vi "FipsAdjacent.vi"() -> (11 "Fips":i32[](array[numeric]))   [LabVIEW 2017] (continued)
KS\"\t20097\t\"Ford County, KS\"\t20057\n\"Kiowa County, KS\"\t20097\t\"Kiowa County, KS\"\t20097\n\"Kiowa County, KS\"\t20097\t\"Pratt County, KS\"\t20151\n\"Labette County, KS\"\t20099\t\"Cherokee County, KS\"\t20021\n\"Labette County, KS\"\t20099\t\"Crawford County, KS\"\t20037\n\"Labette County, KS\"\t20099\t\"Labette County, KS\"\t20099\n\"Labette County, KS\"\t20099\t\"Montgomery County, KS\"\t20125\n\"Labette County, KS\"\t20099\t\"Neosho County, KS\"\t20133\n\"Labette County, KS\"\t20099\t\"Craig County, OK\"\t40035\n\"Labette County, KS\"\t20099\t\"Nowata County, OK\"\t40105\n\"Lane County, KS\"\t20101\t\"Finney County, KS\"\t20055\n\"Lane County, KS\"\t20101\t\"Gove County, KS\"\t20063\n\"Lane County, KS\"\t20101\t\"Lane County, KS\"\t20101\n\"Lane County, KS\"\t20101\t\"Ness County, KS\"\t20135\n\"Lane County, KS\"\t20101\t\"Scott County, KS\"\t20171\n\"Leavenworth County, KS\"\t20103\t\"Atchison County, KS\"\t20005\n\"Leavenworth County, KS\"\t20103\t\"Douglas County, KS\"\t20045\n\"Leavenworth County, KS\"\t20103\t\"Jefferson County, KS\"\t20087\n\"Leavenworth County, KS\"\t20103\t\"Johnson County, KS\"\t20091\n\"Leavenworth County, KS\"\t20103\t\"Leavenworth County, KS\"\t20103\n\"Leavenworth County, KS\"\t20103\t\"Wyandotte County, KS\"\t20209\n\"Leavenworth County, KS\"\t20103\t\"Platte County, MO\"\t29165\n\"Lincoln County, KS\"\t20105\t\"Ellsworth County, KS\"\t20053\n\"Lincoln County, KS\"\t20105\t\"Lincoln County, KS\"\t20105\n\"Lincoln County, KS\"\t20105\t\"Mitchell County, KS\"\t20123\n\"Lincoln County, KS\"\t20105\t\"Osborne County, KS\"\t20141\n\"Lincoln County, KS\"\t20105\t\"Ottawa County, KS\"\t20143\n\"Lincoln County, KS\"\t20105\t\"Russell County, KS\"\t20167\n\"Lincoln County, KS\"\t20105\t\"Saline County, KS\"\t20169\n\"Linn County, KS\"\t20107\t\"Allen County, KS\"\t20001\n\"Linn County, KS\"\t20107\t\"Anderson County, KS\"\t20003\n\"Linn County, KS\"\t20107\t\"Bourbon County, KS\"\t20011\n\"Linn County, KS\"\t20107\t\"Franklin County, KS\"\t20059\n\"Linn County, KS\"\t20107\t\"Linn County, KS\"\t20107\n\"Linn County, KS\"\t20107\t\"Miami County, KS\"\t20121\n\"Linn County, KS\"\t20107\t\"Bates County, MO\"\t29013\n\"Linn County, KS\"\t20107\t\"Vernon County, MO\"\t29217\n\"Logan County, KS\"\t20109\t\"Gove County, KS\"\t20063\n\"Logan County, KS\"\t20109\t\"Logan County, KS\"\t20109\n\"Logan County, KS\"\t20109\t\"Scott County, KS\"\t20171\n\"Logan County, KS\"\t20109\t\"Sherman County, KS\"\t20181\n\"Logan County, KS\"\t20109\t\"Thomas County, KS\"\t20193\n\"Logan County, KS\"\t20109\t\"Wallace County, KS\"\t20199\n\"Logan County, KS\"\t20109\t\"Wichita County, KS\"\t20203\n\"Lyon County, KS\"\t20111\t\"Chase County, KS\"\t20017\n\"Lyon County, KS\"\t20111\t\"Coffey County, KS\"\t20031\n\"Lyon County, KS\"\t20111\t\"Greenwood County, KS\"\t20073\n\"Lyon County, KS\"\t20111\t\"Lyon County, KS\"\t20111\n\"Lyon County, KS\"\t20111\t\"Morris County, KS\"\t20127\n\"Lyon County, KS\"\t20111\t\"Osage County, KS\"\t20139\n\"Lyon County, KS\"\t20111\t\"Wabaunsee County, KS\"\t20197\n\"McPherson County, KS\"\t20113\t\"Dickinson County, KS\"\t20041\n\"McPherson County, KS\"\t20113\t\"Ellsworth County, KS\"\t20053\n\"McPherson County, KS\"\t20113\t\"Harvey County, KS\"\t20079\n\"McPherson County, KS\"\t20113\t\"McPherson County, KS\"\t20113\n\"McPherson County, KS\"\t20113\t\"Marion County, KS\"\t20115\n\"McPherson County, KS\"\t20113\t\"Reno County, KS\"\t20155\n\"McPherson County, KS\"\t20113\t\"Rice County, KS\"\t20159\n\"McPherson County, KS\"\t20113\t\"Saline County, KS\"\t20169\n\"Marion County, KS\"\t20115\t\"Butler County, KS\"\t20015\n\"Marion County, KS\"\t20115\t\"Chase County, KS\"\t20017\n\"Marion County, KS\"\t20115\t\"Dickinson County, KS\"\t20041\n\"Marion County, KS\"\t20115\t\"Harvey County, KS\"\t20079\n\"Marion County, KS\"\t20115\t\"McPherson County, KS\"\t20113\n\"Marion County, KS\"\t20115\t\"Marion County, KS\"\t20115\n\"Marion County, KS\"\t20115\t\"Morris County, KS\"\t20127\n\"Marion County, KS\"\t20115\t\"Saline County, KS\"\t20169\n\"Marshall County, KS\"\t20117\t\"Marshall County, KS\"\t20117\n\"Marshall County, KS\"\t20117\t\"Nemaha County, KS\"\t20131\n\"Marshall County, KS\"\t20117\t\"Pottawatomie County, KS\"\t20149\n\"Marshall County, KS\"\t20117\t\"Riley County, KS\"\t20161\n\"Marshall County, KS\"\t20117\t\"Washington County, KS\"\t20201\n\"Marshall County, KS\"\t20117\t\"Gage County, NE\"\t31067\n\"Marshall County, KS\"\t20117\t\"Pawnee County, NE\"\t31133\n\"Meade County, KS\"\t20119\t\"Clark County, KS\"\t20025\n\"Meade County, KS\"\t20119\t\"Ford County, KS\"\t20057\n\"Meade County, KS\"\t20119\t\"Gray County, KS\"\t20069\n\"Meade County, KS\"\t20119\t\"Haskell County, KS\"\t20081\n\"Meade County, KS\"\t20119\t\"Meade County, KS\"\t20119\n\"Meade County, KS\"\t20119\t\"Seward County, KS\"\t20175\n\"Meade County, KS\"\t20119\t\"Beaver County, OK\"\t40007\n\"Miami County, KS\"\t20121\t\"Anderson County, KS\"\t20003\n\"Miami County, KS\"\t20121\t\"Douglas County, KS\"\t20045\n\"Miami County, KS\"\t20121\t\"Franklin County, KS\"\t20059\n\"Miami County, KS\"\t20121\t\"Johnson County, KS\"\t20091\n\"Miami County, KS\"\t20121\t\"Linn County, KS\"\t20107\n\"Miami County, KS\"\t20121\t\"Miami County, KS\"\t20121\n\"Miami County, KS\"\t20121\t\"Bates County, MO\"\t29013\n\"Miami County, KS\"\t20121\t\"Cass County, MO\"\t29037\n\"Mitchell County, KS\"\t20123\t\"Cloud County, KS\"\t20029\n\"Mitchell County, KS\"\t20123\t\"Jewell County, KS\"\t20089\n\"Mitchell County, KS\"\t20123\t\"Lincoln County, KS\"\t20105\n\"Mitchell County, KS\"\t20123\t\"Mitchell County, KS\"\t20123\n\"Mitchell County, KS\"\t20123\t\"Osborne County, KS\"\t20141\n\"Mitchell County, KS\"\t20123\t\"Ottawa County, KS\"\t20143\n\"Montgomery County, KS\"\t20125\t\"Chautauqua County, KS\"\t20019\n\"Montgomery County, KS\"\t20125\t\"Elk County, KS\"\t20049\n\"Montgomery County, KS\"\t20125\t\"Labette County, KS\"\t20099\n\"Montgomery County, KS\"\t20125\t\"Montgomery County, KS\"\t20125\n\"Montgomery County, KS\"\t20125\t\"Neosho County, KS\"\t20133\n\"Montgomery County, KS\"\t20125\t\"Wilson County, KS\"\t20205\n\"Montgomery County, KS\"\t20125\t\"Nowata County, OK\"\t40105\n\"Montgomery County, KS\"\t20125\t\"Washington County, OK\"\t40147\n\"Morris County, KS\"\t20127\t\"Chase County, KS\"\t20017\n\"Morris County, KS\"\t20127\t\"Dickinson County, KS\"\t20041\n\"Morris County, KS\"\t20127\t\"Geary County, KS\"\t20061\n\"Morris County, KS\"\t20127\t\"Lyon County, KS\"\t20111\n\"Morris County, KS\"\t20127\t\"Marion County, KS\"\t20115\n\"Morris County, KS\"\t20127\t\"Morris County, KS\"\t20127\n\"Morris County, KS\"\t20127\t\"Wabaunsee County, KS\"\t20197\n\"Morton County, KS\"\t20129\t\"Baca County, CO\"\t08009\n\"Morton County, KS\"\t20129\t\"Morton County, KS\"\t20129\n\"Morton County, KS\"\t20129\t\"Stanton County, KS\"\t20187\n\"Morton County, KS\"\t20129\t\"Stevens County, KS\"\t20189\n\"Morton County, KS\"\t20129\t\"Cimarron County, OK\"\t40025\n\"Morton County, KS\"\t20129\t\"Texas County, OK\"\t40139\n\"Nemaha County, KS\"\t20131\t\"Brown County, KS\"\t20013\n\"Nemaha County, KS\"\t20131\t\"Jackson County, KS\"\t20085\n\"Nemaha County, KS\"\t20131\t\"Marshall County, KS\"\t20117\n\"Nemaha County, KS\"\t20131\t\"Nemaha County, KS\"\t20131\n\"Nemaha County, KS\"\t20131\t\"Pottawatomie County, KS\"\t20149\n\"Nemaha County, KS\"\t20131\t\"Pawnee County, NE\"\t31133\n\"Nemaha County, KS\"\t20131\t\"Richardson County, NE\"\t31147\n\"Neosho County, KS\"\t20133\t\"Allen County, KS\"\t20001\n\"Neosho County, KS\"\t20133\t\"Bourbon County, KS\"\t20011\n\"Neosho County, KS\"\t20133\t\"Crawford County, KS\"\t20037\n\"Neosho County, KS\"\t20133\t\"Labette County, KS\"\t20099\n\"Neosho County, KS\"\t20133\t\"Montgomery County, KS\"\t20125\n\"Neosho County, KS\"\t20133\t\"Neosho County, KS\"\t20133\n\"Neosho County, KS\"\t20133\t\"Wilson County, KS\"\t20205\n\"Neosho County, KS\"\t20133\t\"Woodson County, KS\"\t20207\n\"Ness County, KS\"\t20135\t\"Ellis County, KS\"\t20051\n\"Ness County, KS\"\t20135\t\"Finney County, KS\"\t20055\n\"Ness County, KS\"\t20135\t\"Gove County, KS\"\t20063\n\"Ness County, KS\"\t20135\t\"Hodgeman County, KS\"\t20083\n\"Ness County, KS\"\t20135\t\"Lane County, KS\"\t20101\n\"Ness County, KS\"\t20135\t\"Ness County, KS\"\t20135\n\"Ness County, KS\"\t20135\t\"Pawnee County, KS\"\t20145\n\"Ness County, KS\"\t20135\t\"Rush County, KS\"\t20165\n\"Ness County, KS\"\t20135\t\"Trego County, KS\"\t20195\n\"Norton County, KS\"\t20137\t\"Decatur County, KS\"\t20039\n\"Norton County, KS\"\t20137\t\"Graham County, KS\"\t20065\n\"Norton County, KS\"\t20137\t\"Norton County, KS\"\t20137\n\"Norton County, KS\"\t20137\t\"Phillips County, KS\"\t20147\n\"Norton County, KS\"\t20137\t\"Sheridan County, KS\"\t20179\n\"Norton County, KS\"\t20137\t\"Furnas County, NE\"\t31065\n\"Norton County, KS\"\t20137\t\"Harlan County, NE\"\t31083\n\"Osage County, KS\"\t20139\t\"Coffey County, KS\"\t20031\n\"Osage County, KS\"\t20139\t\"Douglas County, KS\"\t20045\n\"Osage County, KS\"\t20139\t\"Franklin County, KS\"\t20059\n\"Osage County, KS\"\t20139\t\"Lyon County, KS\"\t20111\n\"Osage County, KS\"\t20139\t\"Osage County, KS\"\t20139\n\"Osage County, KS\"\t20139\t\"Shawnee County, KS\"\t20177\n\"Osage County, KS\"\t20139\t\"Wabaunsee County, KS\"\t20197\n\"Osborne County, KS\"\t20141\t\"Ellis County, KS\"\t20051\n\"Osborne County, KS\"\t20141\t\"Jewell County, KS\"\t20089\n\"Osborne County, KS\"\t20141\t\"Lincoln County, KS\"\t20105\n\"Osborne County, KS\"\t20141\t\"Mitchell County, KS\"\t20123\n\"Osborne County, KS\"\t20141\t\"Osborne County, KS\"\t20141\n\"Osborne County, KS\"\t20141\t\"Rooks County, KS\"\t20163\n\"Osborne County, KS\"\t20141\t\"Russell County, KS\"\t20167\n\"Osborne County, KS\"\t20141\t\"Smith County, KS\"\t20183\n\"Ottawa County, KS\"\t20143\t\"Clay County, KS\"\t20027\n\"Ottawa County, KS\"\t20143\t\"Cloud County, KS\"\t20029\n\"Ottawa County, KS\"\t20143\t\"Dickinson County, KS\"\t20041\n\"Ottawa County, KS\"\t20143\t\"Lincoln County, KS\"\t20105\n\"Ottawa County, KS\"\t20143\t\"Mitchell County, KS\"\t20123\n\"Ottawa County, KS\"\t20143\t\"Ottawa County, KS\"\t20143\n\"Ottawa County, KS\"\t20143\t\"Saline County, KS\"\t20169\n\"Pawnee County, KS\"\t20145\t\"Barton County, KS\"\t20009\n\"Pawnee County, KS\"\t20145\t\"Edwards County, KS\"\t20047\n\"Pawnee County, KS\"\t20145\t\"Hodgeman County, KS\"\t20083\n\"Pawnee County, KS\"\t20145\t\"Ness County, KS\"\t20135\n\"Pawnee County, KS\"\t20145\t\"Pawnee County, KS\"\t20145\n\"Pawnee County, KS\"\t20145\t\"Rush County, KS\"\t20165\n\"Pawnee County, KS\"\t20145\t\"Stafford County, KS\"\t20185\n\"Phillips County, KS\"\t20147\t\"Graham County, KS\"\t20065\n\"Phillips County, KS\"\t20147\t\"Norton County, KS\"\t20137\n\"Phillips County, KS\"\t20147\t\"Phillips County, KS\"\t20147\n\"Phillips County, KS\"\t20147\t\"Rooks County, KS\"\t20163\n\"Phillips County, KS\"\t20147\t\"Smith County, KS\"\t20183\n\"Phillips County, KS\"\t20147\t\"Franklin County, NE\"\t31061\n\"Phillips County, KS\"\t20147\t\"Harlan County, NE\"\t31083\n\"Pottawatomie County, KS\"\t20149\t\"Jackson County, KS\"\t20085\n\"Pottawatomie County, KS\"\t20149\t\"Marshall County, KS\"\t20117\n\"Pottawatomie County, KS\"\t20149\t\"Nemaha County, KS\"\t20131\n\"Pottawatomie County, KS\"\t20149\t\"Pottawatomie County, KS\"\t20149\n\"Pottawatomie County, KS\"\t20149\t\"Riley County, KS\"\t20161\n\"Pottawatomie County, KS\"\t20149\t\"Shawnee County, KS\"\t20177\n\"Pottawatomie County, KS\"\t20149\t\"Wabaunsee County, KS\"\t20197\n\"Pratt County, KS\"\t20151\t\"Barber County, KS\"\t20007\n\"Pratt County, KS\"\t20151\t\"Edwards County, KS\"\t20047\n\"Pratt County, KS\"\t20151\t\"Kingman County, KS\"\t20095\n\"Pratt County, KS\"\t20151\t\"Kiowa County, KS\"\t20097\n\"Pratt County, KS\"\t20151\t\"Pratt County, KS\"\t20151\n\"Pratt County, KS\"\t20151\t\"Reno County, KS\"\t20155\n\"Pratt County, KS\"\t20151\t\"Stafford County, KS\"\t20185\n\"Rawlins County, KS\"\t20153\t\"Cheyenne County, KS\"\t20023\n\"Rawlins County, KS\"\t20153\t\"Decatur County, KS\"\t20039\n\"Rawlins County, KS\"\t20153\t\"Rawlins County, KS\"\t20153\n\"Rawlins County, KS\"\t20153\t\"Sherman County, KS\"\t20181\n\"Rawlins County, KS\"\t20153\t\"Thomas County, KS\"\t20193\n\"Rawlins County, KS\"\t20153\t\"Dundy County, NE\"\t31057\n\"Rawlins County, KS\"\t20153\t\"Hitchcock County, NE\"\t31087\n\"Rawlins County, KS\"\t20153\t\"Red Willow County, NE\"\t31145\n\"Reno County, KS\"\t20155\t\"Harvey County, KS\"\t20079\n\"Reno County, KS\"\t20155\t\"Kingman County, KS\"\t20095\n\"Reno County, KS\"\t20155\t\"McPherson County, KS\"\t20113\n\"Reno County, KS\"\t20155\t\"Pratt County, KS\"\t20151\n\"Reno County, KS\"\t20155\t\"Reno County, KS\"\t20155\n\"Reno County, KS\"\t20155\t\"Rice County, KS\"\t20159\n\"Reno County, KS\"\t20155\t\"Sedgwick County, KS\"\t20173\n\"Reno County, KS\"\t20155\t\"Stafford County, KS\"\t20185\n\"Republic County, KS\"\t20157\t\"Cloud County, KS\"\t20029\n\"Republic County, KS\"\t20157\t\"Jewell County, KS\"\t20089\n\"Republic County, KS\"\t20157\t\"Republic County, KS\"\t20157\n\"Republic County, KS\"\t20157\t\"Washington County, KS\"\t20201\n\"Republic County, KS\"\t20157\t\"Jefferson County, NE\"\t31095\n\"Republic County, KS\"\t20157\t\"Nuckolls County, NE\"\t31129\n\"Republic County, KS\"\t20157\t\"Thayer County, NE\"\t31169\n\"Rice County, KS\"\t20159\t\"Barton County, KS\"\t20009\n\"Rice County, KS\"\t20159\t\"Ellsworth County, KS\"\t20053\n\"Rice County, KS\"\t20159\t\"McPherson County, KS\"\t20113\n\"Rice County, KS\"\t20159\t\"Reno County, KS\"\t20155\n\"Rice County, KS\"\t20159\t\"Rice County, KS\"\t20159\n\"Rice County, KS\"\t20159\t\"Stafford County, KS\"\t20185\n\"Riley County, KS\"\t20161\t\"Clay County, KS\"\t20027\n\"Riley County, KS\"\t20161\t\"Geary County, KS\"\t20061\n\"Riley County, KS\"\t20161\t\"Marshall County, KS\"\t20117\n\"Riley County, KS\"\t20161\t\"Pottawatomie County, KS\"\t20149\n\"Riley County, KS\"\t20161\t\"Riley County, KS\"\t20161\n\"Riley County, KS\"\t20161\t\"Wabaunsee County, KS\"\t20197\n\"Riley County, KS\"\t20161\t\"Washington County, KS\"\t20201\n\"Rooks County, KS\"\t20163\t\"Ellis County, KS\"\t20051\n\"Rooks County, KS\"\t20163\t\"Graham County, KS\"\t20065\n\"Rooks County, KS\"\t20163\t\"Osborne County, KS\"\t20141\n\"Rooks County, KS\"\t20163\t\"Phillips County, KS\"\t20147\n\"Rooks County, KS\"\t20163\t\"Rooks County, KS\"\t20163\n\"Rooks County, KS\"\t20163\t\"Smith County, KS\"\t20183\n\"Rooks County, KS\"\t20163\t\"Trego County, KS\"\t20195\n\"Rush County, KS\"\t20165\t\"Barton County, KS\"\t20009\n\"Rush County, KS\"\t20165\t\"Ellis County, KS\"\t20051\n\"Rush County, KS\"\t20165\t\"Ness County, KS\"\t20135\n\"Rush County, KS\"\t20165\t\"Pawnee County, KS\"\t20145\n\"Rush County, KS\"\t20165\t\"Rush County, KS\"\t20165\n\"Rush County, KS\"\t20165\t\"Russell County, KS\"\t20167\n\"Russell County, KS\"\t20167\t\"Barton County, KS\"\t20009\n\"Russell County, KS\"\t20167\t\"Ellis County, KS\"\t20051\n\"Russell County, KS\"\t20167\t\"Ellsworth County, KS\"\t20053\n\"Russell County, KS\"\t20167\t\"Lincoln County, KS\"\t20105\n\"Russell County, KS\"\t20167\t\"Osborne County, KS\"\t20141\n\"Russell County, KS\"\t20167\t\"Rush County, KS\"\t20165\n\"Russell County, KS\"\t20167\t\"Russell County, KS\"\t20167\n\"Saline County, KS\"\t20169\t\"Dickinson County, KS\"\t20041\n\"Saline County, KS\"\t20169\t\"Ellsworth County, KS\"\t20053\n\"Saline County, KS\"\t20169\t\"Lincoln County, KS\"\t20105\n\"Saline County, KS\"\t20169\t\"McPherson County, KS\"\t20113\n\"Saline County, KS\"\t20169\t\"Marion County, KS\"\t20115\n\"Saline County, KS\"\t20169\t\"Ottawa County, KS\"\t20143\n\"Saline County, KS\"\t20169\t\"Saline County, KS\"\t20169\n\"Scott County, KS\"\t20171\t\"Finney County, KS\"\t20055\n\"Scott County, KS\"\t20171\t\"Gove County, KS\"\t20063\n\"Scott County, KS\"\t20171\t\"Kearny County, KS\"\t20093\n\"Scott County, KS\"\t20171\t\"Lane County, KS\"\t20101\n\"Scott County, KS\"\t20171\t\"Logan County, KS\"\t20109\n\"Scott County, KS\"\t20171\t\"Scott County, KS\"\t20171\n\"Scott County, KS\"\t20171\t\"Wichita County, KS\"\t20203\n\"Sedgwick County, KS\"\t20173\t\"Butler County, KS\"\t20015\n\"Sedgwick County, KS\"\t20173\t\"Cowley County, KS\"\t20035\n\"Sedgwick County, KS\"\t20173\t\"Harvey County, KS\"\t20079\n\"Sedgwick County, KS\"\t20173\t\"Kingman County, KS\"\t20095\n\"Sedgwick County, KS\"\t20173\t\"Reno County, KS\"\t20155\n\"Sedgwick County, KS\"\t20173\t\"Sedgwick County, KS\"\t20173\n\"Sedgwick County, KS\"\t20173\t\"Sumner County, KS\"\t20191\n\"Seward County, KS\"\t20175\t\"Haskell County, KS\"\t20081\n\"Seward County, KS\"\t20175\t\"Meade County, KS\"\t20119\n\"Seward County, KS\"\t20175\t\"Seward County, KS\"\t20175\n\"Seward County, KS\"\t20175\t\"Stevens County, KS\"\t20189\n\"Seward County, KS\"\t20175\t\"Beaver County, OK\"\t40007\n\"Seward County, KS\"\t20175\t\"Texas County, OK\"\t40139\n\"Shawnee County, KS\"\t20177\t\"Douglas County, KS\"\t20045\n\"Shawnee County, KS\"\t20177\t\"Jackson County, KS\"\t20085\n\"Shawnee County, KS\"\t20177\t\"Jefferson County, KS\"\t20087\n\"Shawnee County, KS\"\t20177\t\"Osage County, KS\"\t20139\n\"Shawnee County, KS\"\t20177\t\"Pottawatomie County, KS\"\t20149\n\"Shawnee County, KS\"\t20177\t\"Shawnee County, KS\"\t20177\n\"Shawnee County, KS\"\t20177\t\"Wabaunsee County, KS\"\t20197\n\"Sheridan County, KS\"\t20179\t\"Decatur County, KS\"\t20039\n\"Sheridan County, KS\"\t20179\t\"Gove County, KS\"\t20063\n\"Sheridan County, KS\"\t20179\t\"Graham County, KS\"\t20065\n\"Sheridan County, KS\"\t20179\t\"Norton County, KS\"\t20137\n\"Sheridan County, KS\"\t20179\t\"Sheridan County, KS\"\t20179\n\"Sheridan County, KS\"\t20179\t\"Thomas County, KS\"\t20193\n\"Sherman County, KS\"\t20181\t\"Kit Carson County, CO\"\t08063\n\"Sherman County, KS\"\t20181\t\"Cheyenne County, KS\"\t20023\n\"Sherman County, KS\"\t20181\t\"Logan County, KS\"\t20109\n\"Sherman County, KS\"\t20181\t\"Rawlins County, KS\"\t20153\n\"Sherman County, KS\"\t20181\t\"Sherman County, KS\"\t20181\n\"Sherman County, KS\"\t20181\t\"Thomas County, KS\"\t20193\n\"Sherman County, KS\"\t20181\t\"Wallace County, KS\"\t20199\n\"Smith County, KS\"\t20183\t\"Jewell County, KS\"\t20089\n\"Smith County, KS\"\t20183\t\"Osborne County, KS\"\t20141\n\"Smith County, KS\"\t20183\t\"Phillips County, KS\"\t20147\n\"Smith County, KS\"\t20183\t\"Rooks County, KS\"\t20163\n\"Smith County, KS\"\t20183\t\"Smith County, KS\"\t20183\n\"Smith County, KS\"\t20183\t\"Franklin County, NE\"\t31061\n\"Smith County, KS\"\t20183\t\"Webster County, NE\"\t31181\n\"Stafford County, KS\"\t20185\t\"Barton County, KS\"\t20009\n\"Stafford County, KS\"\t20185\t\"Edwards County, KS\"\t20047\n\"Stafford County, KS\"\t20185\t\"Pawnee County, KS\"\t20145\n\"Stafford County, KS\"\t20185\t\"Pratt County, KS\"\t20151\n\"Stafford County, KS\"\t20185\t\"Reno County, KS\"\t20155\n\"Stafford County, KS\"\t20185\t\"Rice County, KS\"\t20159\n\"Stafford County, KS\"\t20185\t\"Stafford County, KS\"\t20185\n\"Stanton County, KS\"\t20187\t\"Baca County, CO\"\t08009\n\"Stanton County, KS\"\t20187\t\"Prowers County, CO\"\t08099\n\"Stanton County, KS\"\t20187\t\"Grant County, KS\"\t20067\n\"Stanton County, KS\"\t20187\t\"Hamilton County, KS\"\t20075\n\"Stanton County, KS\"\t20187\t\"Kearny County, KS\"\t20093\n\"Stanton County, KS\"\t20187\t\"Morton County, KS\"\t20129\n\"Stanton County, KS\"\t20187\t\"Stanton County, KS\"\t20187\n\"Stanton County, KS\"\t20187\t\"Stevens County, KS\"\t20189\n\"Stevens County, KS\"\t20189\t\"Grant County, KS\"\t20067\n\"Stevens County, KS\"\t20189\t\"Haskell County, KS\"\t20081\n\"Stevens County, KS\"\t20189\t\"Morton County, KS\"\t20129\n\"Stevens County, KS\"\t20189\t\"Seward County, KS\"\t20175\n\"Stevens County, KS\"\t20189\t\"Stanton County, KS\"\t20187\n\"Stevens County, KS\"\t20189\t\"Stevens County, KS\"\t20189\n\"Stevens County, KS\"\t20189\t\"Texas County, OK\"\t40139\n\"Sumner County, KS\"\t20191\t\"Butler County, KS\"\t20015\n\"Sumner County, KS\"\t20191\t\"Cowley County, KS\"\t20035\n\"Sumner County, KS\"\t20191\t\"Harper County, KS\"\t20077\n\"Sumner County, KS\"\t20191\t\"Kingman County, KS\"\t20095\n\"Sumner County, KS\"\t20191\t\"Sedgwick County, KS\"\t20173\n\"Sumner County, KS\"\t20191\t\"Sumner County, KS\"\t20191\n\"Sumner County, KS\"\t20191\t\"Grant County, OK\"\t40053\n\"Sumner County, KS\"\t20191\t\"Kay County, OK\"\t40071\n\"Thomas County, KS\"\t20193\t\"Decatur County, KS\"\t20039\n\"Thomas County, KS\"\t20193\t\"Gove County, KS\"\t20063\n\"Thomas County, KS\"\t20193\t\"Logan County, KS\"\t20109\n\"Thomas County, KS\"\t20193\t\"Rawlins County, KS\"\t20153\n\"Thomas County, KS\"\t20193\t\"Sheridan County, KS\"\t20179\n\"Thomas County, KS\"\t20193\t\"Sherman County, KS\"\t20181\n\"Thomas County, KS\"\t20193\t\"Thomas County, KS\"\t20193\n\"Trego County, KS\"\t20195\t\"Ellis County, KS\"\t20051\n\"Trego County, KS\"\t20195\t\"Gove County, KS\"\t20063\n\"Trego County, KS\"\t20195\t\"Graham County, KS\"\t20065\n\"Trego County, KS\"\t20195\t\"Ness County, KS\"\t20135\n\"Trego County, KS\"\t20195\t\"Rooks County, KS\"\t20163\n\"Trego County, KS\"\t20195\t\"Trego County, KS\"\t20195\n\"Wabaunsee County, KS\"\t20197\t\"Geary County, KS\"\t20061\n\"Wabaunsee County, KS\"\t20197\t\"Lyon County, KS\"\t20111\n\"Wabaunsee County, KS\"\t20197\t\"Morris County, KS\"\t20127\n\"Wabaunsee County, KS\"\t20197\t\"Osage County, KS\"\t20139\n\"Wabaunsee County, KS\"\t20197\t\"Pottawatomie County, KS\"\t20149\n\"Wabaunsee County, KS\"\t20197\t\"Riley County, KS\"\t20161\n\"Wabaunsee County, KS\"\t20197\t\"Shawnee County, KS\"\t20177\n\"Wabaunsee County, KS\"\t20197\t\"Wabaunsee County, KS\"\t20197\n\"Wallace County, KS\"\t20199\t\"Cheyenne County, CO\"\t08017\n\"Wallace County, KS\"\t20199\t\"Kit Carson County, CO\"\t08063\n\"Wallace County, KS\"\t20199\t\"Greeley County, KS\"\t20071\n\"Wallace County, KS\"\t20199\t\"Logan County, KS\"\t20109\n\"Wallace County, KS\"\t20199\t\"Sherman County, KS\"\t20181\n\"Wallace County, KS\"\t20199\t\"Wallace County, KS\"\t20199\n\"Wallace County, KS\"\t20199\t\"Wichita County, KS\"\t20203\n\"Washington County, KS\"\t20201\t\"Clay County, KS\"\t20027\n\"Washington County, KS\"\t20201\t\"Cloud County, KS\"\t20029\n\"Washington County, KS\"\t20201\t\"Marshall County, KS\"\t20117\n\"Washington County, KS\"\t20201\t\"Republic County, KS\"\t20157\n\"Washington County, KS\"\t20201\t\"Riley County, KS\"\t20161\n\"Washington County, KS\"\t20201\t\"Washington County, KS\"\t20201\n\"Washington County, KS\"\t20201\t\"Gage County, NE\"\t31067\n\"Washington County, KS\"\t20201\t\"Jefferson County, NE\"\t31095\n\"Washington County, KS\"\t20201\t\"Thayer County, NE\"\t31169\n\"Wichita County, KS\"\t20203\t\"Greeley County, KS\"\t20071\n\"Wichita County, KS\"\t20203\t\"Hamilton County, KS\"\t20075\n\"Wichita County, KS\"\t20203\t\"Kearny County, KS\"\t20093\n\"Wichita County, KS\"\t20203\t\"Logan County, KS\"\t20109\n\"Wichita County, KS\"\t20203\t\"Scott County, KS\"\t20171\n\"Wichita County, KS\"\t20203\t\"Wallace County, KS\"\t20199\n\"Wichita County, KS\"\t20203\t\"Wichita County, KS\"\t20203\n\"Wilson County, KS\"\t20205\t\"Allen County, KS\"\t20001\n\"Wilson County, KS\"\t20205\t\"Elk County, KS\"\t20049\n\"Wilson County, KS\"\t20205\t\"Greenwood County, KS\"\t20073\n\"Wilson County, KS\"\t20205\t\"Montgomery County, KS\"\t20125\n\"Wilson County, KS\"\t20205\t\"Neosho County, KS\"\t20133\n\"Wilson County, KS\"\t20205\t\"Wilson County, KS\"\t20205\n\"Wilson County, KS\"\t20205\t\"Woodson County, KS\"\t20207\n\"Woodson County, KS\"\t20207\t\"Allen County, KS\"\t20001\n\"Woodson County, KS\"\t20207\t\"Anderson County, KS\"\t20003\n\"Woodson County, KS\"\t20207\t\"Coffey County, KS\"\t20031\n\"Woodson County, KS\"\t20207\t\"Greenwood County, KS\"\t20073\n\"Woodson County, KS\"\t20207\t\"Neosho County, KS\"\t20133\n\"Woodson County, KS\"\t20207\t\"Wilson County, KS\"\t20205\n\"Woodson County, KS\"\t20207\t\"Woodson County, KS\"\t20207\n\"Wyandotte County, KS\"\t20209\t\"Johnson County, KS\"\t20091\n\"Wyandotte County, KS\"\t20209\t\"Leavenworth County, KS\"\t20103\n\"Wyandotte County, KS\"\t20209\t\"Wyandotte County, KS\"\t20209\n\"Wyandotte County, KS\"\t20209\t\"Clay County, MO\"\t29047\n\"Wyandotte County, KS\"\t20209\t\"Jackson County, MO\"\t29095\n\"Wyandotte County, KS\"\t20209\t\"Platte County, MO\"\t29165\n\"Adair County, KY\"\t21001\t\"Adair County, KY\"\t21001\n\"Adair County, KY\"\t21001\t\"Casey County, KY\"\t21045\n\"Adair County, KY\"\t21001\t\"Cumberland County, KY\"\t21057\n\"Adair County, KY\"\t21001\t\"Green County, KY\"\t21087\n\"Adair County, KY\"\t21001\t\"Metcalfe County, KY\"\t21169\n\"Adair County, KY\"\t21001\t\"Russell County, KY\"\t21207\n\"Adair County, KY\"\t21001\t\"Taylor County, KY\"\t21217\n\"Allen County, KY\"\t21003\t\"Allen County, KY\"\t21003\n\"Allen County, KY\"\t21003\t\"Barren County, KY\"\t21009\n\"Allen County, KY\"\t21003\t\"Monroe County, KY\"\t21171\n\"Allen County, KY\"\t21003\t\"Simpson County, KY\"\t21213\n\"Allen County, KY\"\t21003\t\"Warren County, KY\"\t21227\n\"Allen County, KY\"\t21003\t\"Macon County, TN\"\t47111\n\"Allen County, KY\"\t21003\t\"Sumner County, TN\"\t47165\n\"Anderson County, KY\"\t21005\t\"Anderson County, KY\"\t21005\n\"Anderson County, KY\"\t21005\t\"Franklin County, KY\"\t21073\n\"Anderson County, KY\"\t21005\t\"Mercer County, KY\"\t21167\n\"Anderson County, KY\"\t21005\t\"Nelson County, KY\"\t21179\n\"Anderson County, KY\"\t21005\t\"Shelby County, KY\"\t21211\n\"Anderson County, KY\"\t21005\t\"Spencer County, KY\"\t21215\n\"Anderson County, KY\"\t21005\t\"Washington County, KY\"\t21229\n\"Anderson County, KY\"\t21005\t\"Woodford County, KY\"\t21239\n\"Ballard County, KY\"\t21007\t\"Alexander County, IL\"\t17003\n\"Ballard County, KY\"\t21007\t\"Pulaski County, IL\"\t17153\n\"Ballard County, KY\"\t21007\t\"Ballard County, KY\"\t21007\n\"Ballard County, KY\"\t21007\t\"Carlisle County, KY\"\t21039\n\"Ballard County, KY\"\t21007\t\"McCracken County, KY\"\t21145\n\"Ballard County, KY\"\t21007\t\"Mississippi County, MO\"\t29133\n\"Barren County, KY\"\t21009\t\"Allen County, KY\"\t21003\n\"Barren County, KY\"\t21009\t\"Barren County, KY\"\t21009\n\"Barren County, KY\"\t21009\t\"Edmonson County, KY\"\t21061\n\"Barren County, KY\"\t21009\t\"Hart County, KY\"\t21099\n\"Barren County, KY\"\t21009\t\"Metcalfe County, KY\"\t21169\n\"Barren County, KY\"\t21009\t\"Monroe County, KY\"\t21171\n\"Barren County, KY\"\t21009\t\"Warren County, KY\"\t21227\n\"Bath County, KY\"\t21011\t\"Bath County, KY\"\t21011\n\"Bath County, KY\"\t21011\t\"Bourbon County, KY\"\t21017\n\"Bath County, KY\"\t21011\t\"Fleming County, KY\"\t21069\n\"Bath County, KY\"\t21011\t\"Menifee County, KY\"\t21165\n\"Bath County, KY\"\t21011\t\"Montgomery County, KY\"\t21173\n\"Bath County, KY\"\t21011\t\"Nicholas County, KY\"\t21181\n\"Bath County, KY\"\t21011\t\"Rowan County, KY\"\t21205\n\"Bell County, KY\"\t21013\t\"Bell County, KY\"\t21013\n\"Bell County, KY\"\t21013\t\"Clay County, KY\"\t21051\n\"Bell County, KY\"\t21013\t\"Harlan County, KY\"\t21095\n\"Bell County, KY\"\t21013\t\"Knox County, KY\"\t21121\n\"Bell County, KY\"\t21013\t\"Leslie County, KY\"\t21131\n\"Bell County, KY\"\t21013\t\"Whitley County, KY\"\t21235\n\"Bell County, KY\"\t21013\t\"Claiborne County, TN\"\t47025\n\"Bell County, KY\"\t21013\t\"Lee County, VA\"\t51105\n\"Boone County, KY\"\t21015\t\"Dearborn County, IN\"\t18029\n\"Boone County, KY\"\t21015\t\"Ohio County, IN\"\t18115\n\"Boone County, KY\"\t21015\t\"Switzerland County, IN\"\t18155\n\"Boone County, KY\"\t21015\t\"Boone County, KY\"\t21015\n\"Boone County, KY\"\t21015\t\"Gallatin County, KY\"\t21077\n\"Boone County, KY\"\t21015\t\"Grant County, KY\"\t21081\n\"Boone County, KY\"\t21015\t\"Kenton County, KY\"\t21117\n\"Boone County, KY\"\t21015\t\"Hamilton County, OH\"\t39061\n\"Bourbon County, KY\"\t21017\t\"Bath County, KY\"\t21011\n\"Bourbon County, KY\"\t21017\t\"Bourbon County, KY\"\t21017\n\"Bourbon County, KY\"\t21017\t\"Clark County, KY\"\t21049\n\"Bourbon County, KY\"\t21017\t\"Fayette County, KY\"\t21067\n\"Bourbon County, KY\"\t21017\t\"Harrison County, KY\"\t21097\n\"Bourbon County, KY\"\t21017\t\"Montgomery County, KY\"\t21173\n\"Bourbon County, KY\"\t21017\t\"Nicholas County, KY\"\t21181\n\"Bourbon County, KY\"\t21017\t\"Scott County, KY\"\t21209\n\"Boyd County, KY\"\t21019\t\"Boyd County, KY\"\t21019\n\"Boyd County, KY\"\t21019\t\"Carter County, KY\"\t21043\n\"Boyd County, KY\"\t21019\t\"Greenup County, KY\"\t21089\n\"Boyd County, KY\"\t21019\t\"Lawrence County, KY\"\t21127\n\"Boyd County, KY\"\t21019\t\"Lawrence County, OH\"\t39087\n\"Boyd County, KY\"\t21019\t\"Wayne County, WV\"\t54099\n\"Boyle County, KY\"\t21021\t\"Boyle County, KY\"\t21021\n\"Boyle County, KY\"\t21021\t\"Casey County, KY\"\t21045\n\"Boyle County, KY\"\t21021\t\"Garrard County, KY\"\t21079\n\"Boyle County, KY\"\t21021\t\"Lincoln County, KY\"\t21137\n\"Boyle County, KY\"\t21021\t\"Marion County, KY\"\t21155\n\"Boyle County, KY\"\t21021\t\"Mercer County, KY\"\t21167\n\"Boyle County, KY\"\t21021\t\"Washington County, KY\"\t21229\n\"Bracken County, KY\"\t21023\t\"Bracken County, KY\"\t21023\n\"Bracken County, KY\"\t21023\t\"Harrison County, KY\"\t21097\n\"Bracken County, KY\"\t21023\t\"Mason County, KY\"\t21161\n\"Bracken County, KY\"\t21023\t\"Pendleton County, KY\"\t21191\n\"Bracken County, KY\"\t21023\t\"Robertson County, KY\"\t21201\n\"Bracken County, KY\"\t21023\t\"Brown County, OH\"\t39015\n\"Bracken County, KY\"\t21023\t\"Clermont County, OH\"\t39025\n\"Breathitt County, KY\"\t21025\t\"Breathitt County, KY\"\t21025\n\"Breathitt County, KY\"\t21025\t\"Knott County, KY\"\t21119\n\"Breathitt County, KY\"\t21025\t\"Lee County, KY\"\t21129\n\"Breathitt County, KY\"\t21025\t\"Magoffin County, KY\"\t21153\n\"Breathitt County, KY\"\t21025\t\"Owsley County, KY\"\t21189\n\"Breathitt County, KY\"\t21025\t\"Perry County, KY\"\t21193\n\"Breathitt County, KY\"\t21025\t\"Wolfe County, KY\"\t21237\n\"Breckinridge County, KY\"\t21027\t\"Perry County, IN\"\t18123\n\"Breckinridge County, KY\"\t21027\t\"Breckinridge County, KY\"\t21027\n\"Breckinridge County, KY\"\t21027\t\"Grayson County, KY\"\t21085\n\"Breckinridge County, KY\"\t21027\t\"Hancock County, KY\"\t21091\n\"Breckinridge County, KY\"\t21027\t\"Hardin County, KY\"\t21093\n\"Breckinridge County, KY\"\t21027\t\"Meade County, KY\"\t21163\n\"Breckinridge County, KY\"\t21027\t\"Ohio County, KY\"\t21183\n\"Bullitt County, KY\"\t21029\t\"Bullitt County, KY\"\t21029\n\"Bullitt County, KY\"\t21029\t\"Hardin County, KY\"\t21093\n\"Bullitt County, KY\"\t21029\t\"Jefferson County, KY\"\t21111\n\"Bullitt County, KY\"\t21029\t\"Nelson County, KY\"\t21179\n\"Bullitt County, KY\"\t21029\t\"Spencer County, KY\"\t21215\n\"Butler County, KY\"\t21031\t\"Butler County, KY\"\t21031\n\"Butler County, KY\"\t21031\t\"Edmonson County, KY\"\t21061\n\"Butler County, KY\"\t21031\t\"Grayson County, KY\"\t21085\n\"Butler County, KY\"\t21031\t\"Logan County, KY\"\t21141\n\"Butler County, KY\"\t21031\t\"Muhlenberg County, KY\"\t21177\n\"Butler County, KY\"\t21031\t\"Ohio County, KY\"\t21183\n\"Butler County, KY\"\t21031\t\"Warren County, KY\"\t21227\n\"Caldwell County, KY\"\t21033\t\"Caldwell County, KY\"\t21033\n\"Caldwell County, KY\"\t21033\t\"Christian County, KY\"\t21047\n\"Caldwell County, KY\"\t21033\t\"Crittenden County, KY\"\t21055\n\"Caldwell County, KY\"\t21033\t\"Hopkins County, KY\"\t21107\n\"Caldwell County, KY\"\t21033\t\"Lyon County, KY\"\t21143\n\"Caldwell County, KY\"\t21033\t\"Trigg County, KY\"\t21221\n\"Caldwell County, KY\"\t21033\t\"Webster County, KY\"\t21233\n\"Calloway County, KY\"\t21035\t\"Calloway County, KY\"\t21035\n\"Calloway County, KY\"\t21035\t\"Graves County, KY\"\t21083\n\"Calloway County, KY\"\t21035\t\"Marshall County, KY\"\t21157\n\"Calloway County, KY\"\t21035\t\"Trigg County, KY\"\t21221\n\"Calloway County, KY\"\t21035\t\"Henry County, TN\"\t47079\n\"Calloway County, KY\"\t21035\t\"Stewart County, TN\"\t47161\n\"Campbell County, KY\"\t21037\t\"Campbell County, KY\"\t21037\n\"Campbell County, KY\"\t21037\t\"Kenton County, KY\"\t21117\n\"Campbell County, KY\"\t21037\t\"Pendleton County, KY\"\t21191\n\"Campbell County, KY\"\t21037\t\"Clermont County, OH\"\t39025\n\"Campbell County, KY\"\t21037\t\"Hamilton County, OH\"\t39061\n\"Carlisle County, KY\"\t21039\t\"Ballard County, KY\"\t21007\n\"Carlisle County, KY\"\t21039\t\"Carlisle County, KY\"\t21039\n\"Carlisle County, KY\"\t21039\t\"Graves County, KY\"\t21083\n\"Carlisle County, KY\"\t21039\t\"Hickman County, KY\"\t21105\n\"Carlisle County, KY\"\t21039\t\"McCracken County, KY\"\t21145\n\"Carlisle County, KY\"\t21039\t\"Mississippi County, MO\"\t29133\n\"Carroll County, KY\"\t21041\t\"Jefferson County, IN\"\t18077\n\"Carroll County, KY\"\t21041\t\"Switzerland County, IN\"\t18155\n\"Carroll County, KY\"\t21041\t\"Carroll County, KY\"\t21041\n\"Carroll County, KY\"\t21041\t\"Gallatin County, KY\"\t21077\n\"Carroll County, KY\"\t21041\t\"Henry County, KY\"\t21103\n\"Carroll County, KY\"\t21041\t\"Owen County, KY\"\t21187\n\"Carroll County, KY\"\t21041\t\"Trimble County, KY\"\t21223\n\"Carter County, KY\"\t21043\t\"Boyd County, KY\"\t21019\n\"Carter County, KY\"\t21043\t\"Carter County, KY\"\t21043\n\"Carter County, KY\"\t21043\t\"Elliott County, KY\"\t21063\n\"Carter County, KY\"\t21043\t\"Greenup County, KY\"\t21089\n\"Carter County, KY\"\t21043\t\"Lawrence County, KY\"\t21127\n\"Carter County, KY\"\t21043\t\"Lewis County, KY\"\t21135\n\"Carter County, KY\"\t21043\t\"Rowan County, KY\"\t21205\n\"Casey County, KY\"\t21045\t\"Adair County, KY\"\t21001\n\"Casey County, KY\"\t21045\t\"Boyle County, KY\"\t21021\n\"Casey County, KY\"\t21045\t\"Casey County, KY\"\t21045\n\"Casey County, KY\"\t21045\t\"Lincoln County, KY\"\t21137\n\"Casey County, KY\"\t21045\t\"Marion County, KY\"\t21155\n\"Casey County, KY\"\t21045\t\"Pulaski County, KY\"\t21199\n\"Casey County, KY\"\t21045\t\"Russell County, KY\"\t21207\n\"Casey County, KY\"\t21045\t\"Taylor County, KY\"\t21217\n\"Christian County, KY\"\t21047\t\"Caldwell County, KY\"\t21033\n\"Christian County, KY\"\t21047\t\"Christian County, KY\"\t21047\n\"Christian County, KY\"\t21047\t\"Hopkins County, KY\"\t21107\n\"Christian County, KY\"\t21047\t\"Muhlenberg County, KY\"\t21177\n\"Christian County, KY\"\t21047\t\"Todd County, KY\"\t21219\n\"Christian County, KY\"\t21047\t\"Trigg County, KY\"\t21221\n\"Christian County, KY\"\t21047\t\"Montgomery County, TN\"\t47125\n\"Christian County, KY\"\t21047\t\"Stewart County, TN\"\t47161\n\"Clark County, KY\"\t21049\t\"Bourbon County, KY\"\t21017\n\"Clark County, KY\"\t21049\t\"Clark County, KY\"\t21049\n\"Clark County, KY\"\t21049\t\"Estill County, KY\"\t21065\n\"Clark County, KY\"\t21049\t\"Fayette County, KY\"\t21067\n\"Clark County, KY\"\t21049\t\"Madison County, KY\"\t21151\n\"Clark County, KY\"\t21049\t\"Montgomery County, KY\"\t21173\n\"Clark County, KY\"\t21049\t\"Powell County, KY\"\t21197\n\"Clay County, KY\"\t21051\t\"Bell County, KY\"\t21013\n\"Clay County, KY\"\t21051\t\"Clay County, KY\"\t21051\n\"Clay County, KY\"\t21051\t\"Jackson County, KY\"\t21109\n\"Clay County, KY\"\t21051\t\"Knox County, KY\"\t21121\n\"Clay County, KY\"\t21051\t\"Laurel County, KY\"\t21125\n\"Clay County, KY\"\t21051\t\"Leslie County, KY\"\t21131\n\"Clay County, KY\"\t21051\t\"Owsley County, KY\"\t21189\n\"Clay County, KY\"\t21051\t\"Perry County, KY\"\t21193\n\"Clinton County, KY\"\t21053\t\"Clinton County, KY\"\t21053\n\"Clinton County, KY\"\t21053\t\"Cumberland County, KY\"\t21057\n\"Clinton County, KY\"\t21053\t\"Russell County, KY\"\t21207\n\"Clinton County, KY\"\t21053\t\"Wayne County, KY\"\t21231\n\"Clinton County, KY\"\t21053\t\"Clay County, TN\"\t47027\n\"Clinton County, KY\"\t21053\t\"Pickett County, TN\"\t47137\n\"Crittenden County, KY\"\t21055\t\"Hardin County, IL\"\t17069\n\"Crittenden County, KY\"\t21055\t\"Caldwell County, KY\"\t21033\n\"Crittenden County, KY\"\t21055\t\"Crittenden County, KY\"\t21055\n\"Crittenden County, KY\"\t21055\t\"Livingston County, KY\"\t21139\n\"Crittenden County, KY\"\t21055\t\"Lyon County, KY\"\t21143\n\"Crittenden County, KY\"\t21055\t\"Union County, KY\"\t21225\n\"Crittenden County, KY\"\t21055\t\"Webster County, KY\"\t21233\n\"Cumberland County, KY\"\t21057\t\"Adair County, KY\"\t21001\n\"Cumberland County, KY\"\t21057\t\"Clinton County, KY\"\t21053\n\"Cumberland County, KY\"\t21057\t\"Cumberland County, KY\"\t21057\n\"Cumberland County, KY\"\t21057\t\"Metcalfe County, KY\"\t21169\n\"Cumberland County, KY\"\t21057\t\"Monroe County, KY\"\t21171\n\"Cumberland County, KY\"\t21057\t\"Russell County, KY\"\t21207\n\"Cumberland County, KY\"\t21057\t\"Clay County, TN\"\t47027\n\"Daviess County, KY\"\t21059\t\"Spencer County, IN\"\t18147\n\"Daviess County, KY\"\t21059\t\"Warrick County, IN\"\t18173\n\"Daviess County, KY\"\t21059\t\"Daviess County, KY\"\t21059\n\"Daviess County, KY\"\t21059\t\"Hancock County, KY\"\t21091\n\"Daviess County, KY\"\t21059\t\"Henderson County, KY\"\t21101\n\"Daviess County, KY\"\t21059\t\"McLean County, KY\"\t21149\n\"Daviess County, KY\"\t21059\t\"Ohio County, KY\"\t21183\n\"Edmonson County, KY\"\t21061\t\"Barren County, KY\"\t21009\n\"Edmonson County, KY\"\t21061\t\"Butler County, KY\"\t21031\n\"Edmonson County, KY\"\t21061\t\"Edmonson County, KY\"\t21061\n\"Edmonson County, KY\"\t21061\t\"Grayson County, KY\"\t21085\n\"Edmonson County, KY\"\t21061\t\"Hart County, KY\"\t21099\n\"Edmonson County, KY\"\t21061\t\"Warren County, KY\"\t21227\n\"Elliott County, KY\"\t21063\t\"Carter County, KY\"\t21043\n\"Elliott County, KY\"\t21063\t\"Elliott County, KY\"\t21063\n\"Elliott County, KY\"\t21063\t\"Lawrence County, KY\"\t21127\n\"Elliott County, KY\"\t21063\t\"Morgan County, KY\"\t21175\n\"Elliott County, KY\"\t21063\t\"Rowan County, KY\"\t21205\n\"Estill County, KY\"\t21065\t\"Clark County, KY\"\t21049\n\"Estill County, KY\"\t21065\t\"Estill County, KY\"\t21065\n\"Estill County, KY\"\t21065\t\"Jackson County, KY\"\t21109\n\"Estill County, KY\"\t21065\t\"Lee County, KY\"\t21129\n\"Estill County, KY\"\t21065\t\"Madison County, KY\"\t21151\n\"Estill County, KY\"\t21065\t\"Powell County, KY\"\t21197\n\"Fayette County, KY\"\t21067\t\"Bourbon County, KY\"\t21017\n\"Fayette County, KY\"\t21067\t\"Clark County, KY\"\t21049\n\"Fayette County, KY\"\t21067\t\"Fayette County, KY\"\t21067\n\"Fayette County, KY\"\t21067\t\"Jessamine County, KY\"\t21113\n\"Fayette County, KY\"\t21067\t\"Madison County, KY\"\t21151\n\"Fayette County, KY\"\t21067\t\"Scott County, KY\"\t21209\n\"Fayette County, KY\"\t21067\t\"Woodford County, KY\"\t21239\n\"Fleming County, KY\"\t21069\t\"Bath County, KY\"\t21011\n\"Fleming County, KY\"\t21069\t\"Fleming County, KY\"\t21069\n\"Fleming County, KY\"\t21069\t\"Lewis County, KY\"\t21135\n\"Fleming County, KY\"\t21069\t\"Mason County, KY\"\t21161\n\"Fleming County, KY\"\t21069\t\"Nicholas County, KY\"\t21181\n\"Fleming County, KY\"\t21069\t\"Robertson County, KY\"\t21201\n\"Fleming County, KY\"\t21069\t\"Rowan County, KY\"\t21205\n\"Floyd County, KY\"\t21071\t\"Floyd County, KY\"\t21071\n\"Floyd County, KY\"\t21071\t\"Johnson County, KY\"\t21115\n\"Floyd County, KY\"\t21071\t\"Knott County, KY\"\t21119\n\"Floyd County, KY\"\t21071\t\"Magoffin County, KY\"\t21153\n\"Floyd County, KY\"\t21071\t\"Martin County, KY\"\t21159\n\"Floyd County, KY\"\t21071\t\"Pike County, KY\"\t21195\n\"Franklin County, KY\"\t21073\t\"Anderson County, KY\"\t21005\n\"Franklin County, KY\"\t21073\t\"Franklin County, KY\"\t21073\n\"Franklin County, KY\"\t21073\t\"Henry County, KY\"\t21103\n\"Franklin County, KY\"\t21073\t\"Owen County, KY\"\t21187\n\"Franklin County, KY\"\t21073\t\"Scott County, KY\"\t21209\n\"Franklin County, KY\"\t21073\t\"Shelby County, KY\"\t21211\n\"Franklin County, KY\"\t21073\t\"Woodford County, KY\"\t21239\n\"Fulton County, KY\"\t21075\t\"Fulton County, KY\"\t21075\n\"Fulton
